vi "IFile Read.vi"(8 "error in (no error)":errorcluster, 11 "INIScoreFile in":refnum<class "INIScoreFile.lvclass">) -> (0 "error out":errorcluster, 3 "INIScoreFile out":refnum<class "INIScoreFile.lvclass">)   [LabVIEW 2020, in "INIScoreFile.lvclass"]
uses:
  INIScoreFile.lvclass
  INIScoreFile.lvclass/INIScoreFile.ctl
  ca15bf14-c902-4f7a-81d1-88d36f941a54.vi
  <vilib>/Comparison/Less/Less Functor/Less Functor.lvclass
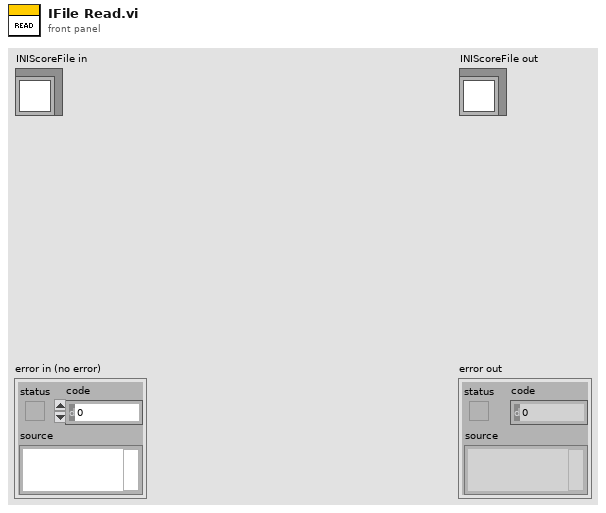
[diagram p1: front panel]
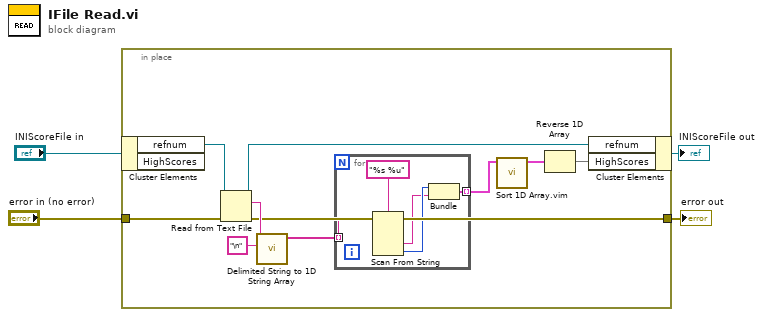
[diagram p0: block diagram]
diagram:
  n1 = in-place {
    in-place-border: "error in (no error)" -> [w13]
    in-place-border: [w8] -> w1
    n2 = in-place-cluster #1("INIScoreFile in") -> ("refnum"=w14:refnum<file>)  [unwired: 1 out]
    n3 = Read from Text File(file (use dialog)=w14, error in=w13) -> (refnum out=w9:refnum<file>, text=w12:string, error out=w8:errorcluster)  [unwired: 2 in, 1 out]
    n4 = call <vilib>:"Delimited String to 1D String Array.vi"("delimiter"="\n", "delimited string"=w12) -> ("string array"=w10:string[])  [unwired: 9 in]
    n5 = for {
      tunnel: w10 -> [w19] mode=indexing
      tunnel: [w17] -> w7 mode=indexing
      n6 = Scan From String(format string="%s %u", input string=w19) -> (output 1=w15:string, output 2=w16:u32)  [unwired: 4 in, 3 out]
      n7 = Bundle(w16, w15) -> (w17:cluster{u32, string})  [unwired: 1 in]
    }
    n8 = call "Sort 1D Array.vim"("unsorted array"=w7) -> ("sorted array"=w6:cluster{u32, string}[])  [unwired: 10 in]
    n9 = Reverse 1D Array(array=w6) -> (reversed array=w5:cluster{u32, string}[])
    n10 = in-place-cluster #1("refnum"=w9, "HighScores"=w5) -> (→"INIScoreFile out":refnum<class "INIScoreFile.lvclass">)
  }
  "error out" <- w1
